vi "Main.vi"(8 "error in":errorcluster, 11 "gRPC Read in":refnum<class "gRPC Read.lvclass">) -> (0 "error out":errorcluster, 3 "gRPC Read out":refnum<class "gRPC Read.lvclass">)   [LabVIEW 2019, in "gRPC Client (template.proto).lvlib" / "gRPC Read.lvclass"]
doc: "The <b>Queued Message Handler</b> of the Worker that owns this VI."
uses:
  gRPC Read.lvclass
  Initialization Data.ctl
  Response Cases.ctl
  <vilib>/addons/_Workers/Library/Case Label.ctl
  <vilib>/gRPC/LabVIEW gRPC Library/Shared/grpcId.ctl
  gRPC Read.lvclass/gRPC Read.ctl
  rql_Read Incoming Data from Server.ctl
  <vilib>/gRPC/LabVIEW gRPC Library/grpc-lvsupport-release.lvlib
  <vilib>/addons/_Workers/Library/Workers.lvlib
  Generated_client/Generated_client.lvlib
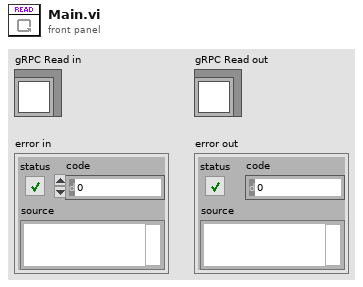
[diagram p1: front panel]
types:
  T1 = typedef "gRPC Client (template.proto).lvlib/gRPC Read.lvclass/Initialization Data.ctl" = cluster{"Response Cases":T2, "Call ID":T4}
  T2 = typedef "gRPC Client (template.proto).lvlib/gRPC Read.lvclass/Response Cases.ctl" = cluster{"Receive Incoming gRPC Data":T3, "Connection Lost":T3}
  T3 = typedef "Workers.lvlib/Case Label.ctl" = string
  T4 = typedef "grpc-lvsupport-release.lvlib/grpcId.ctl" = u64
  T5 = typedef "gRPC Client (template.proto).lvlib/gRPC Read.lvclass/rql_Read Incoming Data from Server.ctl" = cluster{"Placeholder":string}
  T6 = typedef "Generated_client.lvlib/w4lvgrpc_ToClient.ctl" = cluster{"w4lvgrpc_ToClient_payload":refnum<class "w4lvgrpc_ToClient_payload.lvclass">}
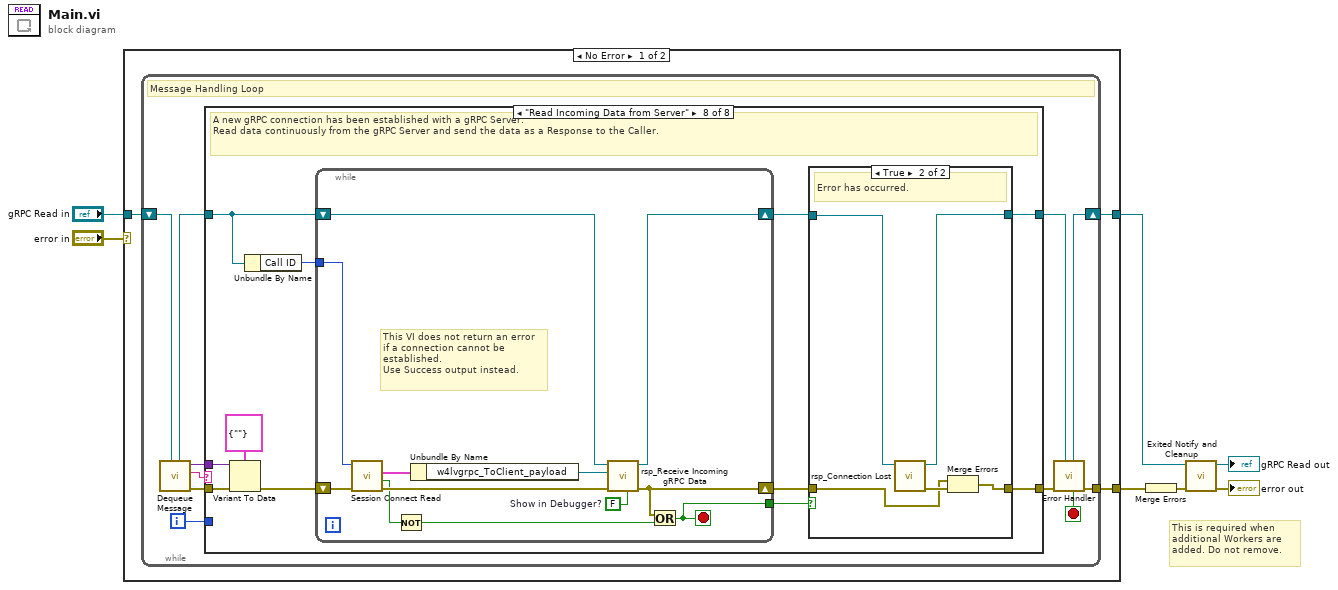
[diagram p0: block diagram]
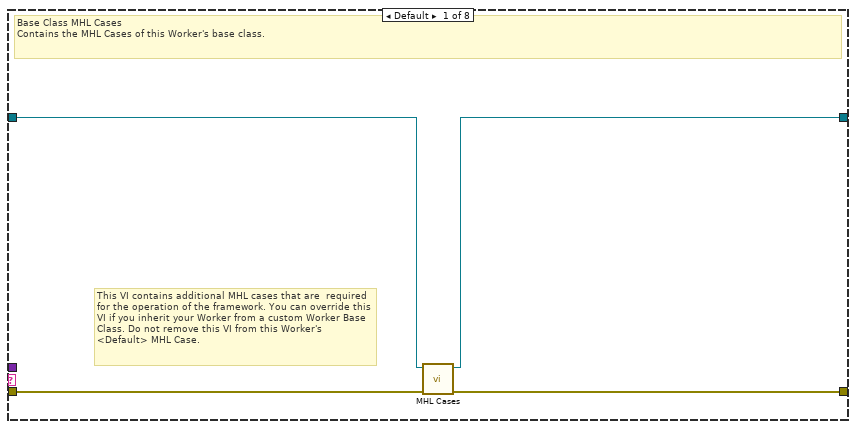
[diagram p2: hidden frame]
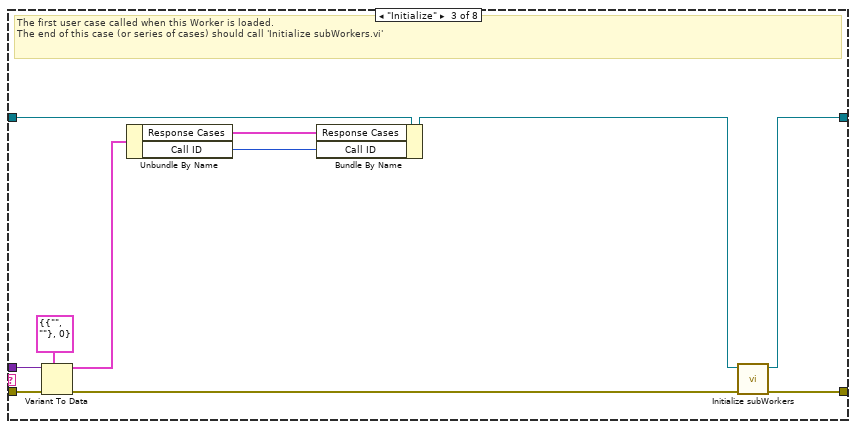
[diagram p4: hidden frame]
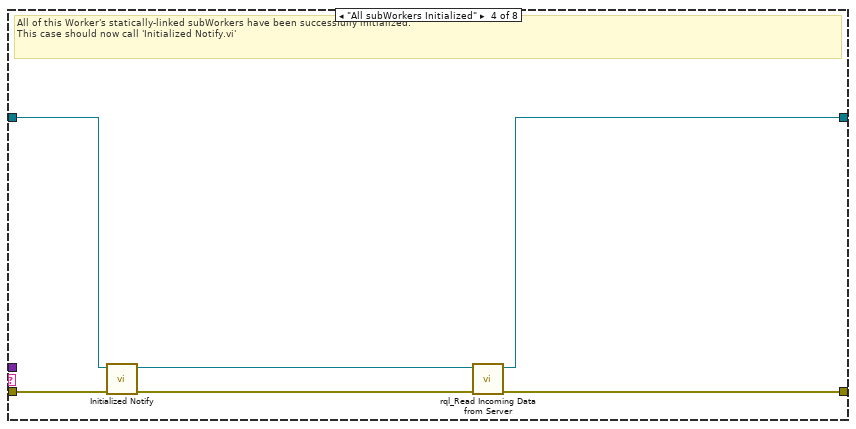
[diagram p5: hidden frame]
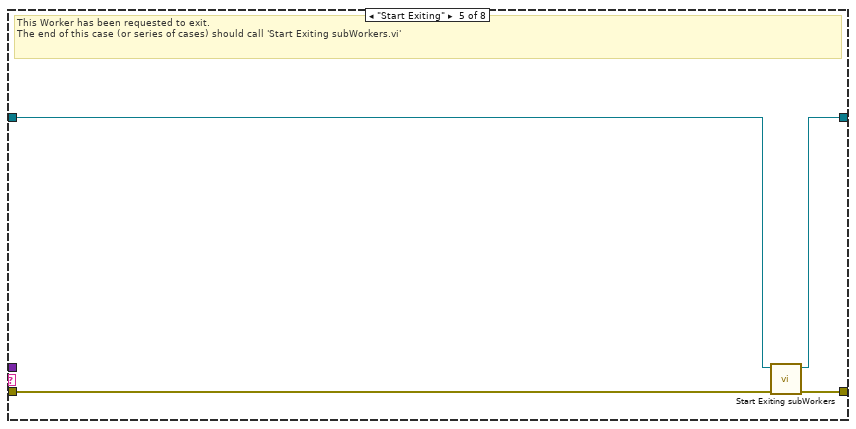
[diagram p6: hidden frame]
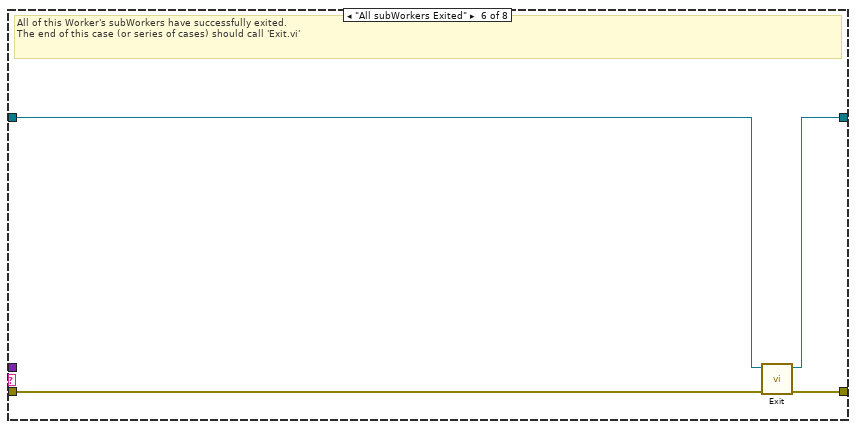
[diagram p7: hidden frame]
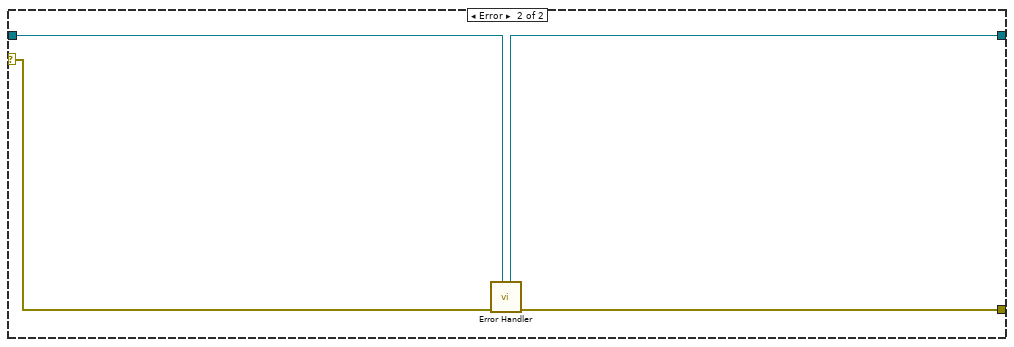
[diagram p10: hidden frame]
diagram:
  # "This is required when additional Workers are added. Do not remove."
  n1 = case shown="No Error" "error in" {
    tunnel: "gRPC Read in" -> [w8 w86]
    tunnel: [w10 w87] -> w6
    tunnel: [w9 w85] -> w7
    selector: "error in" -> [_ w88]
    frame No Error {
      n2 = while {
        shift-right: [w19] -> w9
        shift-left: w8 -> [w21]
        tunnel: [w20] -> w10
        i -> [w12]
        stop <- w13 stop-if-true
        # "Message Handling Loop"
        n3 = call-dynamic "Dequeue Message.vi"("Worker"=w21) -> ("error out"=w18:errorcluster, "Case out"=w14:string, "Data out"=w11:variant, "Worker out"=w16:refnum<class "gRPC Read.lvclass">)  [unwired: 6 in, 1 out]
        n4 = case "Worker MHL Case Structure (DO NOT CHANGE LABEL NAME)" shown="\"Read Incoming Data from Server\"" w14 {
          tunnel: w18 -> [w25 w26 w36 w44 w45 w52 w54 w65]
          tunnel: [w24 w26 w38 w41 w48 w51 w54 w57] -> w17
          tunnel: w16 -> [w23 w27 w35 w42 w46 w50 w53 w59]
          tunnel: [w22 w27 w37 w39 w47 w49 w53 w58] -> w15
          tunnel: w12 -> [_ _ _ _ _ _ _ _]
          tunnel: w11 -> [_ _ w33 _ _ _ _ w63]
          frame Default {
            # "This VI contains additional MHL cases that are  required for the operation of the framework. You can override this VI if you inherit your Worker from a custom Worker Base Class. Do not remove this VI from this Worker's <Default> MHL Case."
            # "Base Class MHL Cases\nContains the MHL Cases of this Worker's base class."
            n5 = call-dynamic "MHL Cases.vi"("error in"=w25, "Worker in"=w23) -> ("error out"=w24:errorcluster, "Worker out"=w22:refnum<class "gRPC Read.lvclass">)  [unwired: 8 in]
          }
          frame "------------ FRAMEWORK CASES -----------" {
            # "Start of Workers Framework Cases"
          }
          frame "Initialize" {
            # "The first user case called when this Worker is loaded.\nThe end of this case (or series of cases) should call 'Initialize subWorkers.vi'"
            n6 = Variant To Data(error in=w36, type=T1 {"Response Cases"={"Receive Incoming gRPC Data"="", "Connection Lost"=""}, "Call ID"=0} ("Cluster"), Variant=w33) -> (data=w31:T1, error out=w34:errorcluster)
            n7 = Unbundle By Name(w31) -> ("Response Cases"=w30:T2, "Call ID"=w28:T4)
            n8 = Bundle By Name(cluster=w35, "Response Cases"=w30, "Call ID"=w28) -> (w32:refnum<class "gRPC Read.lvclass">)
            n9 = call-dynamic "Initialize subWorkers.vi"("error in"=w34, "Worker"=w32) -> ("error out"=w38:errorcluster, "dup Worker out"=w37:refnum<class "gRPC Read.lvclass">)  [unwired: 8 in]
          }
          frame "All subWorkers Initialized" {
            # "All of this Worker's statically-linked subWorkers have been successfully initialized.\nThis case should now call 'Initialized Notify.vi'"
            n10 = call-dynamic "Initialized Notify.vi"("error in"=w44, "Worker"=w42) -> ("error out"=w43:errorcluster, "dup Worker out"=w40:refnum<class "gRPC Read.lvclass">)  [unwired: 8 in]
            n11 = call "rql_Read Incoming Data from Server.vi"("error in"=w43, "gRPC Read in"=w40) -> ("error out"=w41:errorcluster, "dup gRPC Read out"=w39:refnum<class "gRPC Read.lvclass">)  [unwired: 8 in]
          }
          frame "Start Exiting" {
            # "This Worker has been requested to exit. \nThe end of this case (or series of cases) should call 'Start Exiting subWorkers.vi'"
            n12 = call-dynamic "Start Exiting subWorkers.vi"("error_in"=w45, "Worker"=w46) -> ("error out"=w48:errorcluster, "dup Worker out"=w47:refnum<class "gRPC Read.lvclass">)  [unwired: 8 in]
          }
          frame "All subWorkers Exited" {
            # "All of this Worker's subWorkers have successfully exited. \nThe end of this case (or series of cases) should call 'Exit.vi'"
            n13 = call-dynamic "Exit.vi"("error_in"=w52, "Worker"=w50) -> ("error out"=w51:errorcluster, "dup Worker out"=w49:refnum<class "gRPC Read.lvclass">)  [unwired: 8 in]
          }
          frame "------------- LOCAL API CASES -------------" {
            # "Start of Workers Local API Cases"
          }
          frame "Read Incoming Data from Server" {
            # "A new gRPC connection has been established with a gRPC Server.\nRead data continuously from the gRPC Server and send the data as a Response to the Caller."
            n14 = Variant To Data(error in=w65, type=T5 {"Placeholder"=""} ("Data"), Variant=w63) -> (error out=w60:errorcluster)  [unwired: 1 out]
            n15 = Unbundle By Name(w59) -> ("Call ID"=w56:T4)
            n16 = while {
              shift-right: [w74] -> w61
              shift-left: w60 -> [w81]
              shift-right: [w82] -> w62
              shift-left: w59 -> [w78]
              tunnel: w56 -> [w76]
              tunnel: [w73] -> w55
              stop <- w73 stop-if-true
              w83 = FALSE  # Show in Debugger?
              # "This VI does not return an error\nif a connection cannot be \nestablished.\nUse Success output instead."
              n17 = call "Session Connect Read.vi"("error in"=w81, "Call ID in"=w76) -> ("error out"=w80:errorcluster, "Success"=w77:bool, "Response Data"=w79:T6)  [unwired: 6 in, 1 out]
              n18 = Not(x=w77) -> (.not. x?=w75:bool)
              n19 = Unbundle By Name(w79) -> ("w4lvgrpc_ToClient_payload"=w84:refnum<class "w4lvgrpc_ToClient_payload.lvclass">)
              n20 = call "rsp_Receive Incoming gRPC Data.vi"("Show in Debugger?"=w83, "error in"=w80, "Data in"=w84, "gRPC Read in"=w78) -> ("error out"=w74:errorcluster, "gRPC Read in"=w82:refnum<class "gRPC Read.lvclass">)  [unwired: 6 in]
              n21 = Or(x=w74, y=w75) -> (x .or. y?=w73:bool)
            }
            n22 = case shown="True" w55 {
              tunnel: [w66 w70] -> w57
              tunnel: [w67 w71] -> w58
              tunnel: w62 -> [w67 w68]
              tunnel: w61 -> [w66 w69]
              frame False {
              }
              frame True {
                # "Error has occurred."
                n23 = call "rsp_Connection Lost.vi"("gRPC Read in"=w68) -> ("error out"=w72:errorcluster, "dup gRPC Read out"=w71:refnum<class "gRPC Read.lvclass">)  [unwired: 9 in]
                n24 = Merge Errors(w69, w72) -> (w70:errorcluster)
              }
            }
          }
        }
        n25 = call-dynamic "Error Handler.vi"("Worker"=w15, "error_in"=w17) -> ("error out"=w20:errorcluster, "Stop Loop"=w13:bool, "Worker out"=w19:refnum<class "gRPC Read.lvclass">)  [unwired: 7 in]
      }
    }
    frame Error {
      n26 = call-dynamic "Error Handler.vi"("Worker"=w86, "error_in"=w88) -> ("error out"=w87:errorcluster, "Worker out"=w85:refnum<class "gRPC Read.lvclass">)  [unwired: 7 in, 1 out]
    }
  }
  n27 = Merge Errors(w6) -> (w3:errorcluster)
  n28 = call-dynamic "Exited Notify and Cleanup.vi"("error_in"=w3, "Worker"=w7) -> ("error out"=→"error out":errorcluster, "dup Worker out"=→"gRPC Read out":refnum<class "gRPC Read.lvclass">)  [unwired: 8 in]
